vi "autofocus.vi"(3 "Focus function":enum16{"Std dev", "Edges std dev"}(ring)=enum."Edges std dev", 4 "initial focal step":dbl=4.0, 5 "dynamic scope variables":T1) -> (0 "Number of captures":i32, 1 "Focus position":dbl, 2 "dynamic scope variables out":T1)   [LabVIEW 2011]
uses:
  typedefs/dynamic_data.ctl
  <vilib>/vision/Image Controls.llb/IMAQ Image.ctl
  typedefs/autofocus_states.ctl
panel:
  in  "Direction":bool
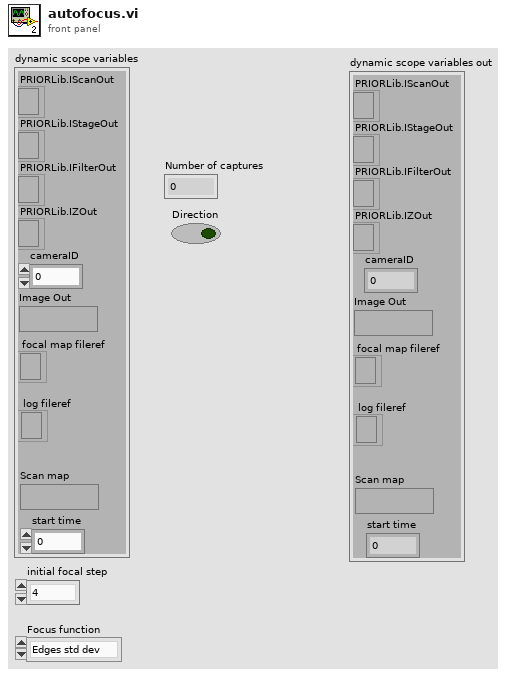
[diagram p1: front panel]
types:
  T1 = typedef "dynamic_data.ctl" = cluster{"PRIORLib.IScanOut":refnum<k7>, "PRIORLib.IStageOut":refnum<k7>, "PRIORLib.IFilterOut":refnum<k7>, "PRIORLib.IZOut":refnum<k7>, "cameraID":u32, "Image Out":T2, "focal map fileref":refnum<file>, "Scan map":T2, "start time":u32, "log fileref":refnum<file>}
  T2 = typedef "IMAQ Image.ctl" = refnum<image>
  T3 = typedef "autofocus_states.ctl" = enum16{"Count cells", "Find direction", "Focus", "Finalize"}
  T4 = cluster{"Mean Value":sgl, "Standard Variation":sgl, "Minimal Value":sgl, "Maximal Value":sgl, "Area (calibrated)":sgl, "Area (pixels)":u32, "%":sgl, "Calibration Valid":bool}
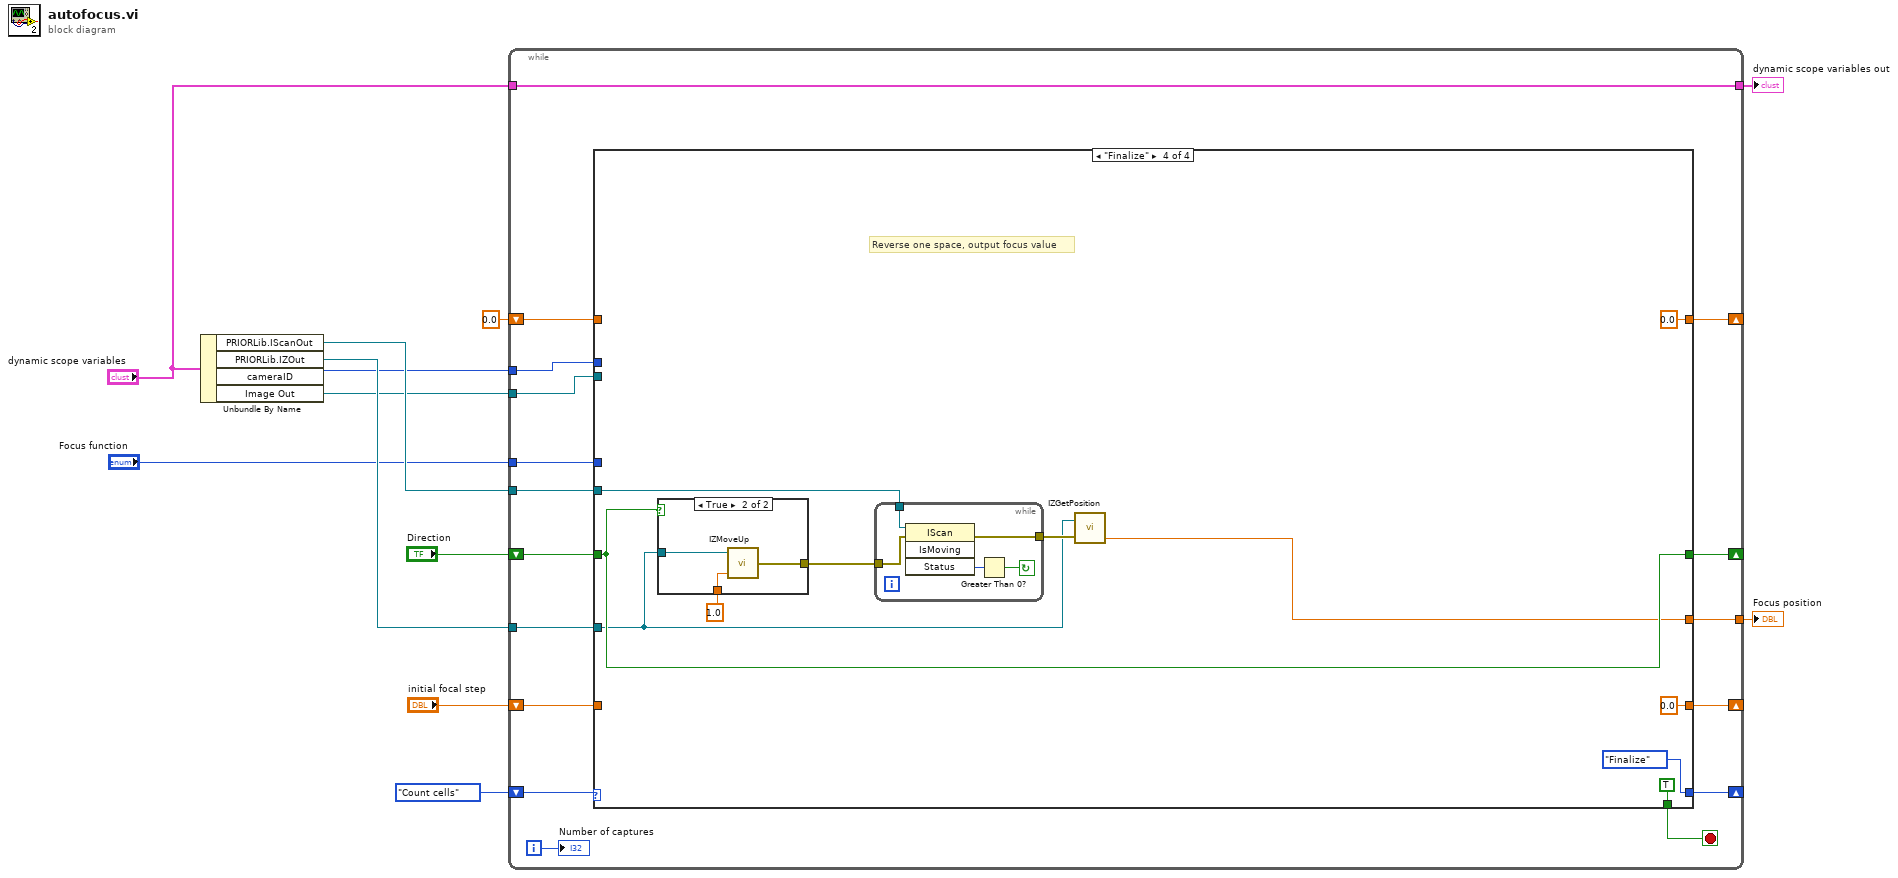
[diagram p0: block diagram]
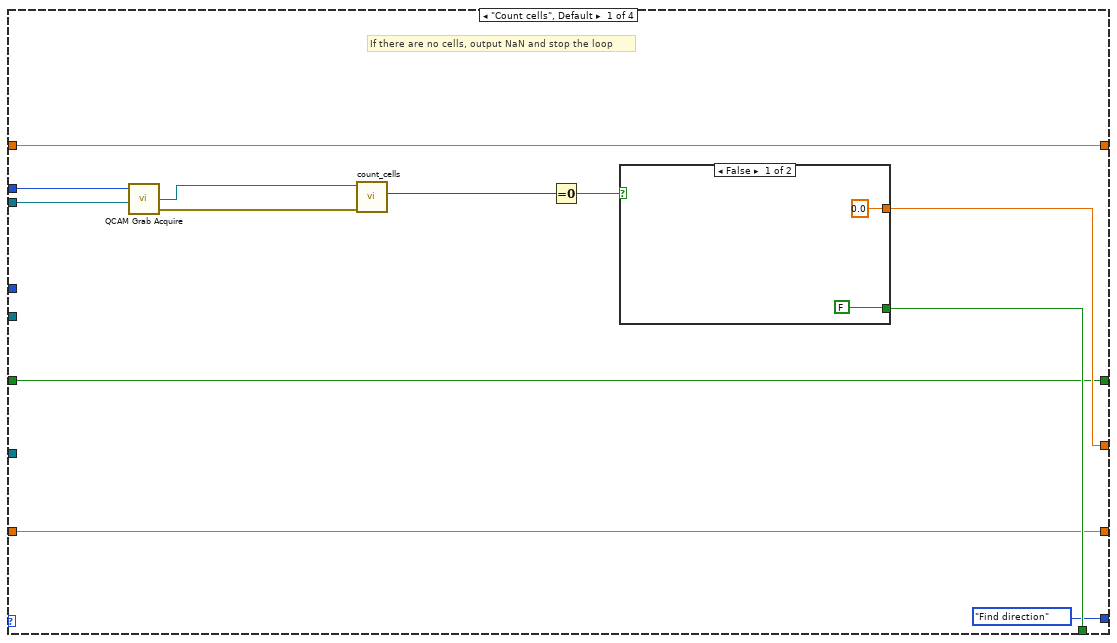
[diagram p2: hidden frame]
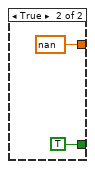
[diagram p3: hidden frame]
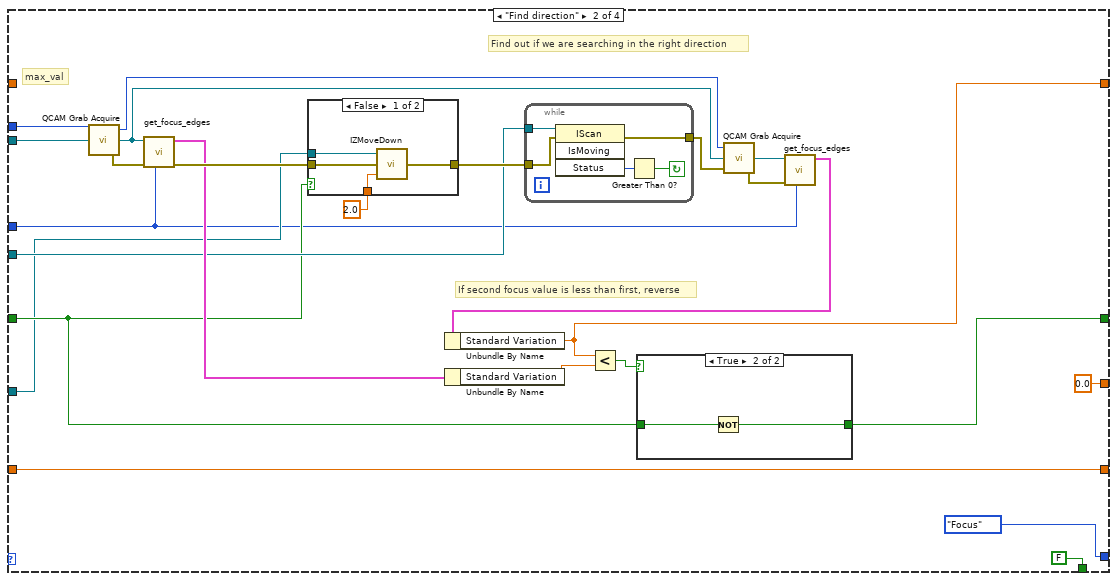
[diagram p4: hidden frame]
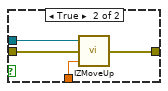
[diagram p6: hidden frame]
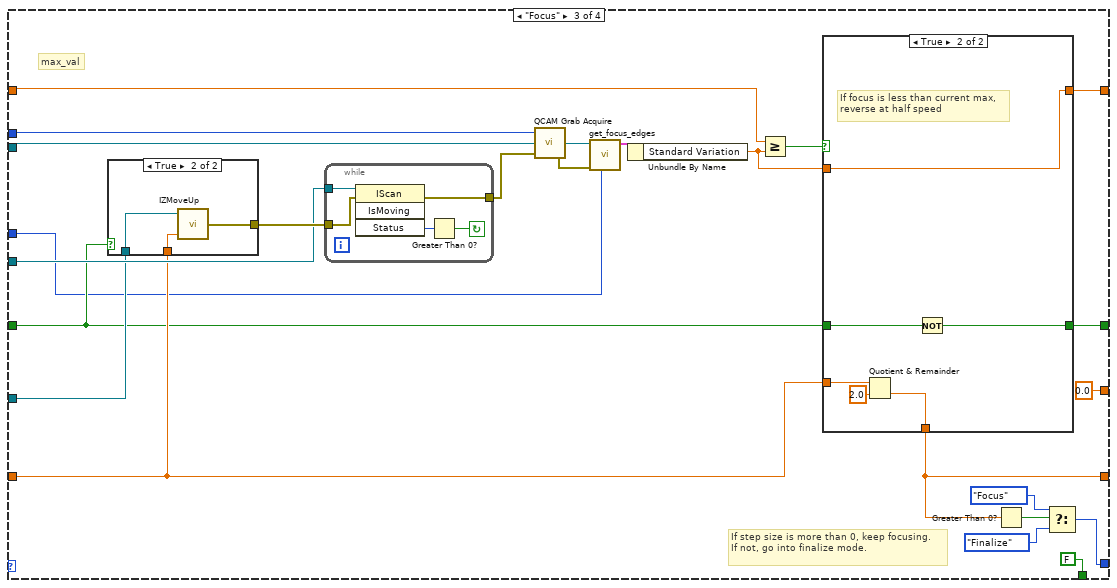
[diagram p7: hidden frame]
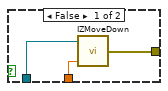
[diagram p8: hidden frame]
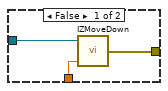
[diagram p10: hidden frame]
diagram:
  n1 = Unbundle By Name("dynamic scope variables") -> ("PRIORLib.IScanOut"=w6:refnum<k7>, "PRIORLib.IZOut"=w7:refnum<k7>, "cameraID"=w5:u32, "Image Out"=w4:T2)
  n2 = while {
    tunnel: w4 -> [w19]
    tunnel: w5 -> [w20]
    tunnel: w6 -> [w26]
    tunnel: w7 -> [w15]
    shift-right: [w27] -> _
    shift-left: autofocus_states."Count cells" -> [w28]
    shift-right: [w25] -> _
    shift-left: sgl 0.0 ("Maximal Value") -> [w24]
    shift-right: [w21] -> _
    shift-left: "initial focal step" -> [w22]
    tunnel: [w18] -> w9
    shift-right: [w16] -> _
    shift-left: "Direction" -> [w17]
    tunnel: "dynamic scope variables" -> [w14]
    tunnel: [w14] -> w2
    tunnel: "Focus function" -> [w13]
    i -> [w29]
    stop <- w23 stop-if-true
    n3 = case shown="\"Finalize\"" w28 {
      tunnel: [autofocus_states."Find direction" autofocus_states."Focus" w98 autofocus_states."Finalize"] -> w27
      tunnel: w15 -> [_ w48 w95 w132]
      tunnel: w26 -> [_ w58 w96 w140]
      tunnel: w19 -> [w40 w60 w105 _]
      tunnel: w20 -> [w41 w59 w106 _]
      tunnel: [w35 w49 w101 sgl 0.0 ("Standard Variation")] -> w25
      tunnel: w24 -> [w35 _ w107 _]
      tunnel: [w37 FALSE FALSE TRUE] -> w23
      tunnel: w22 -> [w33 w53 w93 _]
      tunnel: [w33 w53 w94 0.0 ("focal step")] -> w21
      tunnel: [w36 0.0 ("ZPos") 0.0 ("ZPos") w131] -> w18
      tunnel: w17 -> [w34 w52 w89 w133]
      tunnel: [w34 w51 w88 w133] -> w16
      tunnel: w13 -> [_ w46 w87 _]
      frame "Count cells", Default {
        # "If there are no cells, output NaN and stop the loop"
        n4 = call <userlib>:"QCAM Grab Acquire.vi"("Image"=w40, "cameraId"=w41) -> ("error out"=w30:errorcluster, "Image Out"=w31:T2)  [unwired: 1 in, 1 out]
        n5 = call "count_cells.vi"("error in"=w30, "Image In"=w31) -> ("Number of Particles (Particle Analysis 1)"=w39:i32)  [unwired: 6 in, 3 out]
        n6 = Equal To 0?(x=w39) -> (x = 0?=w38:bool)
        n7 = case shown="False" w38 {
          tunnel: [FALSE TRUE] -> w37
          tunnel: [0.0 ("ZPos") nan ("ZPos")] -> w36
          frame False {
          }
          frame True {
          }
        }
      }
      frame "Find direction" {
        # "max_val"
        # "If second focus value is less than first, reverse"
        # "Find out if we are searching in the right direction"
        n8 = call <userlib>:"QCAM Grab Acquire.vi"("Image"=w60, "cameraId"=w59) -> ("error out"=w62:errorcluster, "Image Out"=w70:T2, "cameraId out"=w57:u32)  [unwired: 1 in]
        n9 = call "get_focus_edges.vi"("Focus function"=w46, "error in (no error)"=w62, "Image in"=w70) -> ("error out"=w65:errorcluster, "Global Report"=w61:T4)  [unwired: 7 in]
        n10 = case shown="False" w52 {
          tunnel: [w81 w86] -> w63
          tunnel: 2.0 ("Distance") -> [w82 w85]
          tunnel: w65 -> [w80 w83]
          tunnel: w48 -> [w79 w84]
          frame False {
            n11 = call "IZMoveDown.vi"("Distance"=w82, "error in (no error)"=w80, "PRIORLib.IZIn"=w79) -> ("error out"=w81:errorcluster)  [unwired: 2 out]
          }
          frame True {
            n12 = call "IZMoveUp.vi"("Distance"=w85, "error in (no error)"=w83, "PRIORLib.IZIn"=w84) -> ("error out"=w86:errorcluster)  [unwired: 2 out]
          }
        }
        n13 = Unbundle By Name(w61) -> ("Standard Variation"=w50:sgl)
        n14 = while {
          tunnel: w63 -> [w76]
          tunnel: [w75] -> w69
          tunnel: w58 -> [w74]
          stop <- w77 continue-if-true
          n15 = invoke class="IScan" method="IsMoving"(reference=w74, error in=w76) -> (error out=w75:errorcluster, "Status"=w78:i32)  [unwired: 2 in, 2 out]
          n16 = Greater Than 0?(x=w78) -> (x > 0?=w77:bool)
        }
        n17 = call <userlib>:"QCAM Grab Acquire.vi"("error in (no error)"=w69, "Image"=w70, "cameraId"=w57) -> ("error out"=w68:errorcluster, "Image Out"=w67:T2)  [unwired: 1 out]
        n18 = call "get_focus_edges.vi"("Focus function"=w46, "error in (no error)"=w68, "Image in"=w67) -> ("Global Report"=w66:T4)  [unwired: 7 in, 1 out]
        n19 = Unbundle By Name(w66) -> ("Standard Variation"=w49:sgl)
        n20 = Less?(x=w49, y=w50) -> (x < y?=w56:bool)
        n21 = case shown="True" w56 {
          tunnel: w52 -> [w71 w73]
          tunnel: [w71 w72] -> w51
          frame False {
          }
          frame True {
            n22 = Not(x=w73) -> (.not. x?=w72:bool)
          }
        }
      }
      frame "Focus" {
        # "If step size is more than 0, keep focusing.\nIf not, go into finalize mode."
        # "max_val"
        n23 = case shown="True" w89 {
          tunnel: [w117 w121] -> w104
          tunnel: w93 -> [w118 w120]
          tunnel: w95 -> [w116 w119]
          frame False {
            n24 = call "IZMoveDown.vi"("Distance"=w118, "PRIORLib.IZIn"=w116) -> ("error out"=w117:errorcluster)  [unwired: 1 in, 2 out]
          }
          frame True {
            n25 = call "IZMoveUp.vi"("Distance"=w120, "PRIORLib.IZIn"=w119) -> ("error out"=w121:errorcluster)  [unwired: 1 in, 2 out]
          }
        }
        n26 = while {
          tunnel: w104 -> [w113]
          tunnel: [w112] -> w103
          tunnel: w96 -> [w111]
          stop <- w114 continue-if-true
          n27 = invoke class="IScan" method="IsMoving"(reference=w111, error in=w113) -> (error out=w112:errorcluster, "Status"=w115:i32)  [unwired: 2 in, 2 out]
          n28 = Greater Than 0?(x=w115) -> (x > 0?=w114:bool)
        }
        n29 = call <userlib>:"QCAM Grab Acquire.vi"("error in (no error)"=w103, "Image"=w105, "cameraId"=w106) -> ("error out"=w109:errorcluster, "Image Out"=w110:T2)  [unwired: 1 out]
        n30 = call "get_focus_edges.vi"("Focus function"=w87, "error in (no error)"=w109, "Image in"=w110) -> ("Global Report"=w108:T4)  [unwired: 7 in, 1 out]
        n31 = Unbundle By Name(w108) -> ("Standard Variation"=w100:sgl)
        n32 = Greater Or Equal?(x=w107, y=w100) -> (x >= y?=w102:bool)
        n33 = case shown="True" w102 {
          tunnel: [w124 w125] -> w101
          tunnel: w100 -> [w124 w125]
          tunnel: [w123 w126] -> w94
          tunnel: w93 -> [w123 w129]
          tunnel: w89 -> [w122 w128]
          tunnel: [w122 w127] -> w88
          frame False {
            # "If current focus is new max,\nupdate max and continue"
          }
          frame True {
            # "If focus is less than current max,\nreverse at half speed"
            n34 = Quotient & Remainder(x=w129, y=2.0) -> (floor(x/y)=w126:dbl)  [unwired: 1 out]
            n35 = Not(x=w128) -> (.not. x?=w127:bool)
          }
        }
        n36 = Greater Than 0?(x=w94) -> (x > 0?=w99:bool)
        n37 = Select(t=autofocus_states."Focus", s=w99, f=autofocus_states."Finalize") -> (s? t:f=w98:T3)
      }
      frame "Finalize" {
        # "Reverse one space, output focus value"
        n38 = case shown="True" w133 {
          tunnel: [w148 w152] -> w141
          tunnel: 1.0 ("focal step") -> [w149 w151]
          tunnel: w132 -> [w147 w150]
          frame False {
            n39 = call "IZMoveDown.vi"("Distance"=w149, "PRIORLib.IZIn"=w147) -> ("error out"=w148:errorcluster)  [unwired: 1 in, 2 out]
          }
          frame True {
            n40 = call "IZMoveUp.vi"("Distance"=w151, "PRIORLib.IZIn"=w150) -> ("error out"=w152:errorcluster)  [unwired: 1 in, 2 out]
          }
        }
        n41 = while {
          tunnel: w141 -> [w144]
          tunnel: [w143] -> w134
          tunnel: w140 -> [w142]
          stop <- w145 continue-if-true
          n42 = invoke class="IScan" method="IsMoving"(reference=w142, error in=w144) -> (error out=w143:errorcluster, "Status"=w146:i32)  [unwired: 2 in, 2 out]
          n43 = Greater Than 0?(x=w146) -> (x > 0?=w145:bool)
        }
        n44 = call "IZGetPosition.vi"("PRIORLib.IZIn"=w132, "error in (no error)"=w134) -> ("ZPos"=w131:dbl)  [unwired: 2 out]
      }
    }
    "Number of captures" <- w29
  }
  "Focus position" <- w9
  "dynamic scope variables out" <- w2
